vi "Show Variables.vi"(8 "error in (no error)":errorcluster, 11 "Python Protocol in":refnum<class "Python Protocol.lvclass">) -> (0 "error out":errorcluster, 3 "Python Protocol out":refnum<class "Python Protocol.lvclass">)   [LabVIEW 2013, in "Python Protocol.lvlib" / "Python Protocol.lvclass"]
uses:
  Python Protocol.lvclass
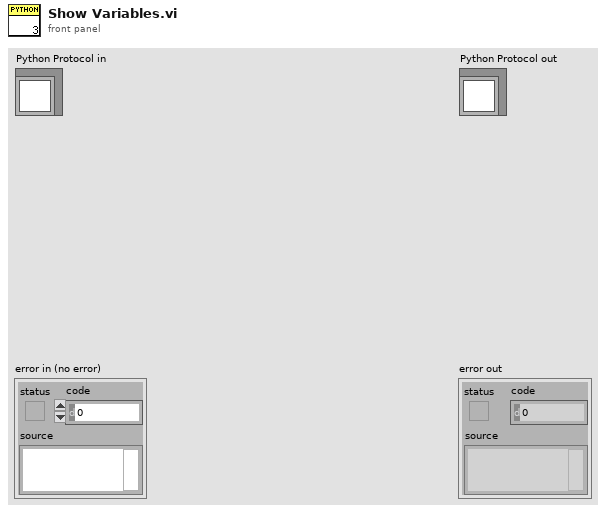
[diagram p1: front panel]
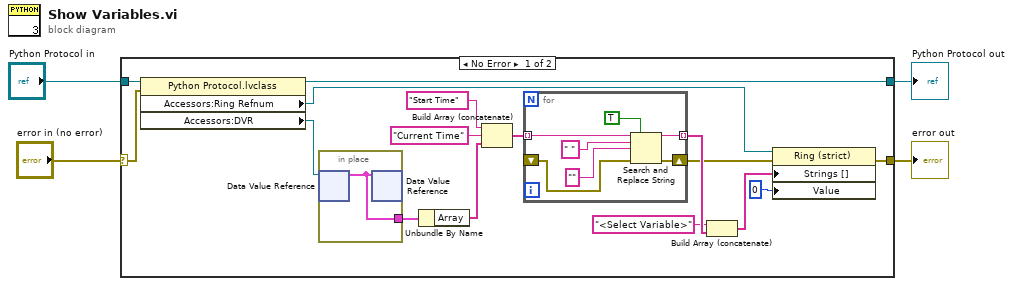
[diagram p0: block diagram]
diagram:
  n1 = case shown="No Error" "error in (no error)" {
    selector: "error in (no error)" -> [w5 w30]
    tunnel: [w6 w30] -> w3
    tunnel: [w19 w29] -> w1
    tunnel: "Python Protocol in" -> [w20 w29]
    frame No Error {
      n2 = property class="Python Protocol.lvclass"(reference=w20, error in=w5) -> (reference out=w19:refnum<class "Python Protocol.lvclass">, "Accessors:Ring Refnum"=w8:refnum<vi>, "Accessors:DVR"=w9:refnum<data-value>)  [unwired: 1 out]
      n3 = in-place {
        in-place-border: [w28] -> w17
        n4 = in-place-dvr #1(w9) -> (w28:cluster{"Array":string[], "Variant":variant})  [unwired: 1 out]
        n5 = in-place-dvr #1(w28) -> ()  [unwired: 2 out]
      }
      n6 = Unbundle By Name(w17) -> ("Array"=w14:string[])
      n7 = Build Array (concatenate)("Start Time" ("element"), "Current Time", w14) -> (w13:string[])
      n8 = for {
        tunnel: w13 -> [w26] mode=indexing
        shift-right: [w22] -> w7
        shift-left: _ -> [w27]
        tunnel: [w21] -> w12 mode=indexing
        n9 = Search and Replace String(replace all?=TRUE ("replace all? (F)"), input string=w26, search string=" ", replace string="" ("replace string (\"\")"), error in=w27) -> (result string=w21:string, error out=w22:errorcluster)  [unwired: 3 in, 2 out]
      }
      n10 = Build Array (concatenate)("<Select Variable>", w12) -> (w10:string[])
      n11 = property class="Ring (strict)"(reference=w8, error in=w7, "Strings []"=w10, "Value"=u16 0) -> (error out=w6:errorcluster)  [unwired: 1 out]
    }
    frame Error {
    }
  }
  "error out" <- w3
  "Python Protocol out" <- w1
